vi "test-DiffOdometry.vi"() -> ()   [LabVIEW 2019]
uses:
  PathExecution_Library/POSE.ctl
  PathExecution_Library/TRANSLATION.ctl
  PathExecution_Library/ROTATION.ctl
  PathExecution_Library/Conv_AngleDegrees_Heading.vi
  PathExecution_Library/PathExecution_Library.lvlib
panel:
  in  "Next Step":bool
  out "ROTATION":T1
  out "HeadingDegrees":dbl
  out "Dist Meters":dbl
  out "CurrentRelativePose":T2
  in  "Reset":bool
  in  "Gyro-Deg":dbl
  in  "Dist Avg":dbl
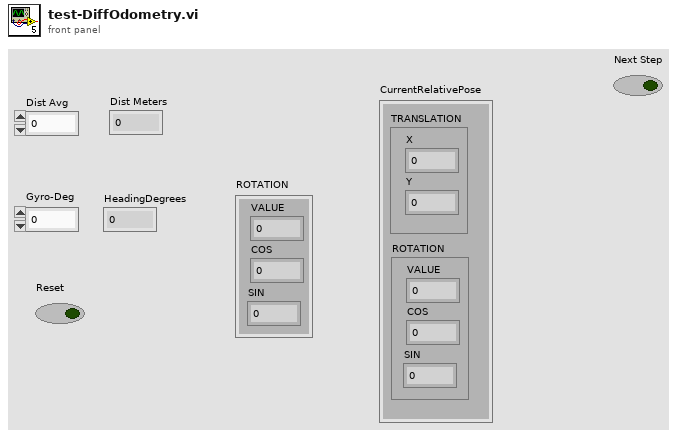
[diagram p1: front panel]
types:
  T1 = typedef "PathExecution_Library.lvlib/ROTATION.ctl" = cluster{"VALUE":dbl, "COS":dbl, "SIN":dbl}
  T2 = typedef "PathExecution_Library.lvlib/POSE.ctl" = cluster{"TRANSLATION":T3, "ROTATION":T1}
  T3 = typedef "PathExecution_Library.lvlib/TRANSLATION.ctl" = cluster{"X":dbl, "Y":dbl}
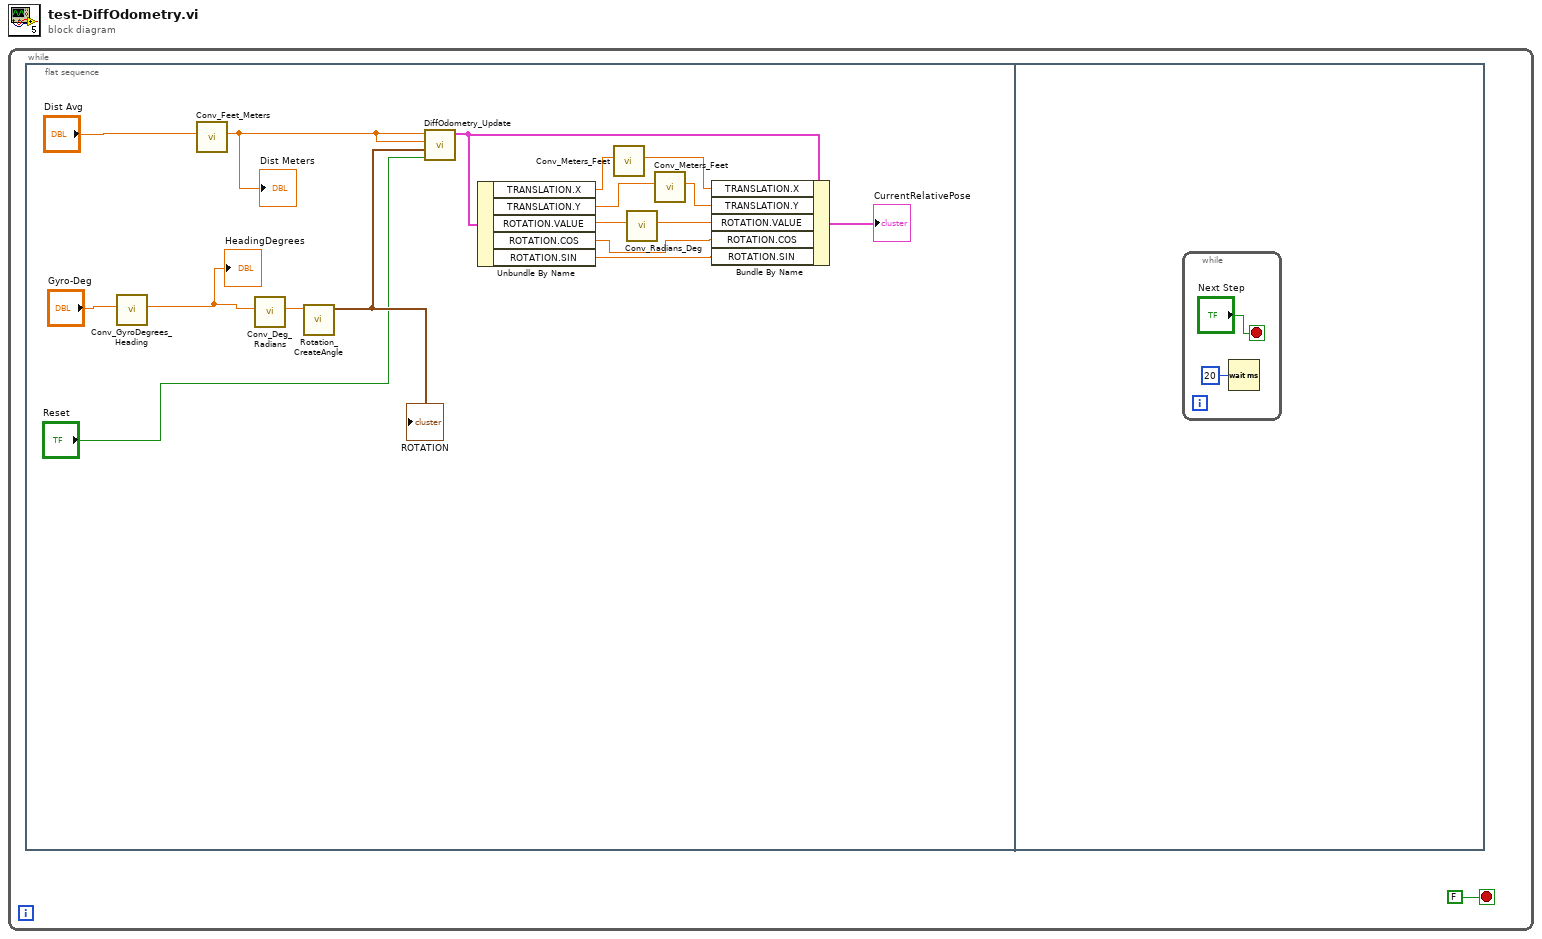
[diagram p0: block diagram]
diagram:
  n1 = while {
    stop <- FALSE stop-if-true
    n2 = flat-sequence {
      frame #0 {
        n3 = call "Conv_GyroDegrees_Heading.vi"("GyroDegrees"="Gyro-Deg") -> ("HeadingDegrees"=w3:dbl)  [unwired: 10 in]
        "HeadingDegrees" <- w3
        n4 = call "Conv_Feet_Meters.vi"("Feet"="Dist Avg") -> ("Meters"=w4:dbl)  [unwired: 10 in]
        "Dist Meters" <- w4
        n5 = call "Conv_Deg_Radians.vi"("Degress"=w3) -> ("Radians"=w2:dbl)  [unwired: 10 in]
        n6 = call "Rotation_CreateAngle.vi"("Angle"=w2) -> ("ROTATION"=w9:T1)  [unwired: 10 in]
        "ROTATION" <- w9
        n7 = call "DiffOdometry_Update.vi"("Reset"="Reset", "Heading"=w9, "RightDistance"=w4, "LeftDistance"=w4) -> ("CurrentRelativePose"=w18:T2)  [unwired: 7 in]
        n8 = Unbundle By Name(w18) -> ("TRANSLATION.X"=w16:dbl, "TRANSLATION.Y"=w15:dbl, "ROTATION.VALUE"=w17:dbl, "ROTATION.COS"=w13:dbl, "ROTATION.SIN"=w12:dbl)
        n9 = call "Conv_Meters_Feet.vi"("Meters"=w16) -> ("Feet"=w10:dbl)  [unwired: 10 in]
        n10 = call "Conv_Radians_Deg.vi"("Radians"=w17) -> ("Degrees"=w14:dbl)  [unwired: 10 in]
        n11 = call "Conv_Meters_Feet.vi"("Meters"=w15) -> ("Feet"=w11:dbl)  [unwired: 10 in]
        n12 = Bundle By Name(cluster=w18, "TRANSLATION.X"=w10, "TRANSLATION.Y"=w11, "ROTATION.VALUE"=w14, "ROTATION.COS"=w13, "ROTATION.SIN"=w12) -> (→"CurrentRelativePose":T2)
      }
      frame #1 {
        n13 = while {
          stop <- "Next Step" stop-if-true
          n14 = Wait (ms)(milliseconds to wait=u32 20) -> ()  [unwired: 1 out]
        }
      }
    }
  }
